vi "ErrorHandler2.vi"(8 "error in":errorcluster, 11 "StringIn":string) -> (0 "output cluster":errorcluster, 2 "ErrorMessage":bool, 3 "StringOut":string)   [LabVIEW 2017]
uses:
  LV_Unicorn.lvlib
panel:
  out "ErrorCode":i32 format="%02x"
  out "OperationCode":i32 format="%02x"
  out "Addres":i32 format="%02x"
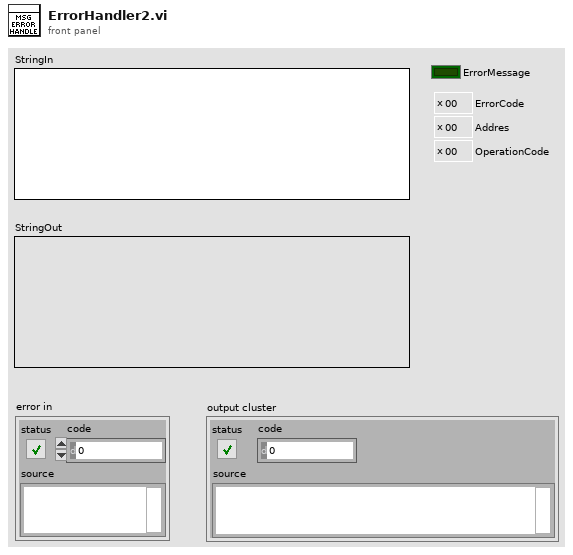
[diagram p1: front panel]
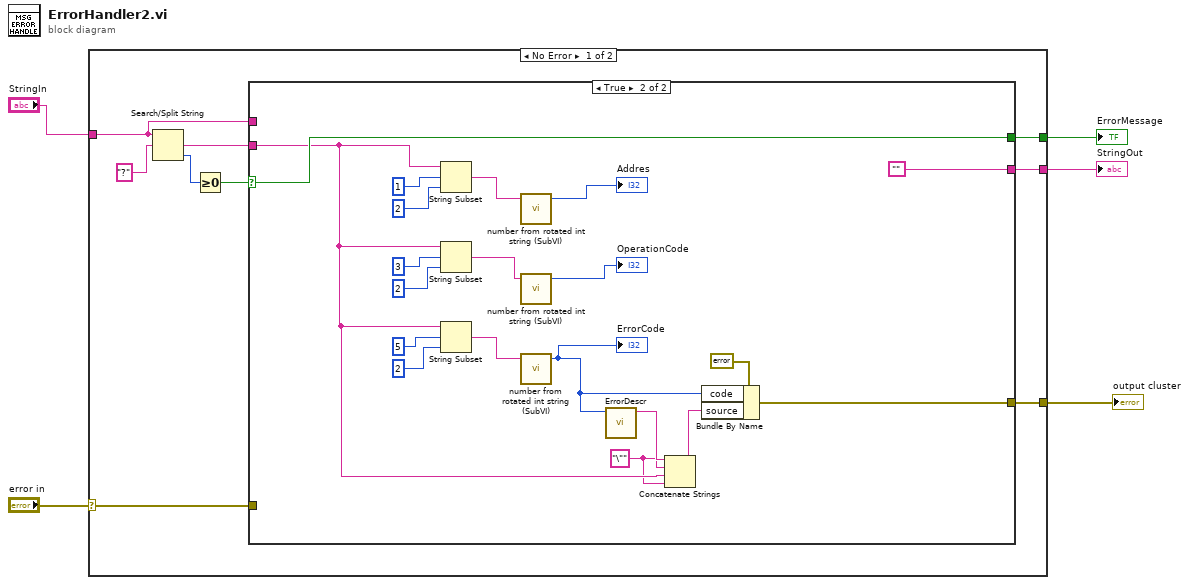
[diagram p0: block diagram]
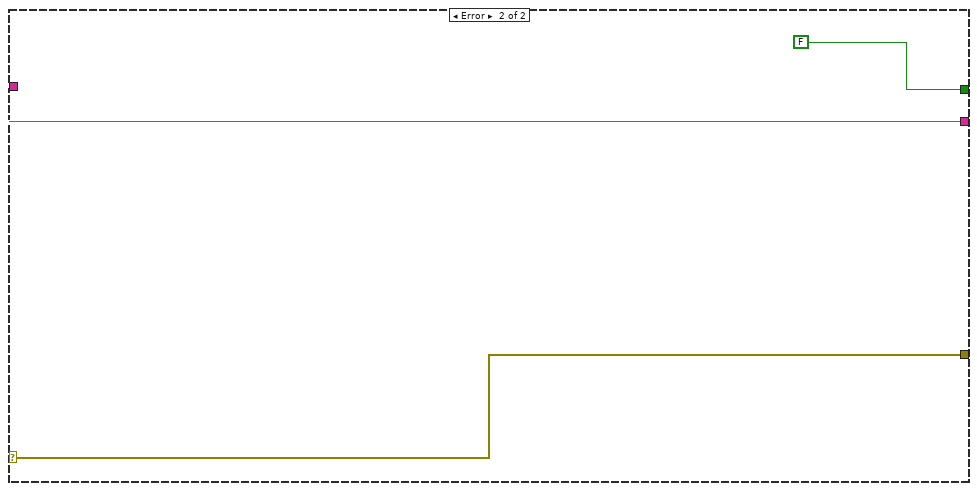
[diagram p3: hidden frame]
diagram:
  n1 = case shown="No Error" "error in" {
    selector: "error in" -> [w9 w40]
    tunnel: [w13 w40] -> w5
    tunnel: [w8 FALSE] -> w3
    tunnel: [w7 w38] -> w2
    tunnel: "StringIn" -> [w6 w38]
    frame No Error {
      n2 = Search/Split String(string=w6, search string/char (-)="?") -> (match + rest of string=w12:string, offset of match=w11:i32)  [unwired: 1 in, 1 out]
      n3 = Greater Or Equal To 0?(x=w11) -> (x >= 0?=w10:bool)
      n4 = case shown="True" w10 {
        selector: w10 -> [w16 w24]
        tunnel: [w17 w25] -> w13
        tunnel: w12 -> [_ w20]
        tunnel: w9 -> [w17 _]
        tunnel: [w16 w24] -> w8
        tunnel: [w15 ""] -> w7
        tunnel: w6 -> [w15 _]
        frame False {
        }
        frame True {
          w19 = "\"" ("string")
          n5 = String Subset(string=w20, offset (0)=1, length (rest)=2 ("length (rest)")) -> (substring=w35:string)
          n6 = String Subset(string=w20, offset (0)=3, length (rest)=2 ("length (rest)")) -> (substring=w31:string)
          n7 = String Subset(string=w20, offset (0)=5, length (rest)=2 ("length (rest)")) -> (substring=w27:string)
          n8 = call "number from rotated int string (SubVI).vi"("String"=w35) -> ("rotated int number"=→"Addres":i32)  [unwired: 2 in, 2 out]
          n9 = call "number from rotated int string (SubVI).vi"("String"=w31) -> ("rotated int number"=→"OperationCode":i32)  [unwired: 2 in, 2 out]
          n10 = call "number from rotated int string (SubVI).vi"("String"=w27) -> ("rotated int number"=w22:i32)  [unwired: 2 in, 2 out]
          "ErrorCode" <- w22
          n11 = call "ErrorDescr.vi"("ErrorCode"=w22) -> ("Desc"=w21:string)  [unwired: 10 in]
          n12 = Concatenate Strings(w21, w19, w20, w19) -> (w18:string)
          n13 = Bundle By Name(cluster=errorcluster {"status"=TRUE, "code"=0, "source"=""} ("error constant"), "code"=w22, "source"=w18) -> (w25:errorcluster)
        }
      }
    }
    frame Error {
    }
  }
  "output cluster" <- w5
  "ErrorMessage" <- w3
  "StringOut" <- w2
